vi "AdaptToInputs.vi"(0 "XRef":T25, 1 "Term Types":T22, 2 "State In":T2={"BlockNodeState"={"Terminal Data"=[], "Instance Name"="", "Type Name"="", "Draw Style"=0, "Connector Pane Pattern"=0, "Flags"=0, "Grown Terminal List Order"=[], "Image"={"image type"=0, "image depth"=0, "image"=[], "mask"=[], "colors"=[], "Rectangle"={"left"=0, "top"=0, "right"=0, "bottom"=0}}}, "stateInfo"={"Data storage parameters"={"Name"="", "Format"="TDM", "Connection string"="", "use default"=TRUE}, "Object type"="root", "Selected properties"=[], "Object definitions"=[], "Refnum input wired"=enum."<none>", "Parent object type"="", "Parent object child property"="", "Channel options"=enum."Replace values at index", "PendingCommand"=enum."<none>", "Node style"=enum."Classic", "Only child objects"=FALSE, "TermSpecs"=[], "objectTypeWired"="", "Dynamic format"=FALSE, "Overwrite options"=enum."open or create", "Parameters"=variant, "Format"="", "Node type"=enum."UPDATE", "ImplicitExplicit"=enum."explicit", "Channel type"=enum."Waveform", "Use object with same name"=FALSE, "Show channel terminal"=FALSE, "LabVIEW Version"="", "DataTerminals"=enum."Express", "Size to text"=FALSE, "selected nodes in"=[]}} {"BlockNodeState"."Draw Style" items=["FunctionBlock", "ExpressVI", "Variable", "Elemental I/O", "32x32 Icon", "FunctionBlockCompact"]; "BlockNodeState"."Terminal Data"."Terminal Flags" format="%.0b"}) -> (14 "Reply":T20, 15 "State Out":T2={"BlockNodeState"={"Terminal Data"=[], "Instance Name"="", "Type Name"="", "Draw Style"=0, "Connector Pane Pattern"=0, "Flags"=0, "Grown Terminal List Order"=[], "Image"={"image type"=0, "image depth"=0, "image"=[], "mask"=[], "colors"=[], "Rectangle"={"left"=0, "top"=0, "right"=0, "bottom"=0}}}, "stateInfo"={"Data storage parameters"={"Name"="", "Format"="TDM", "Connection string"="", "use default"=TRUE}, "Object type"="root", "Selected properties"=[], "Object definitions"=[], "Refnum input wired"=enum."<none>", "Parent object type"="", "Parent object child property"="", "Channel options"=enum."Replace values at index", "PendingCommand"=enum."<none>", "Node style"=enum."Classic", "Only child objects"=FALSE, "TermSpecs"=[], "objectTypeWired"="", "Dynamic format"=FALSE, "Overwrite options"=enum."open or create", "Parameters"=variant, "Format"="", "Node type"=enum."UPDATE", "ImplicitExplicit"=enum."explicit", "Channel type"=enum."Waveform", "Use object with same name"=FALSE, "Show channel terminal"=FALSE, "LabVIEW Version"="", "DataTerminals"=enum."Express", "Size to text"=FALSE, "selected nodes in"=[]}} {"BlockNodeState"."Draw Style" items=["FunctionBlock", "ExpressVI", "Variable", "Elemental I/O", "32x32 Icon", "FunctionBlockCompact"]; "BlockNodeState"."Terminal Data"."Terminal Flags" format="%.0b"})   [LabVIEW 2017, in "Open Data Storage.xnode"]
uses:
  <vilib>/Platform/storage/lvStorage.llb/xStorage/Open Data Storage/Open Data Storage.xnode
  <vilib>/XNodeSupport/XNodeXNodeRef.ctl
  <vilib>/XNodeSupport/XNodeTermTypeIDPairs.ctl
  <vilib>/XNodeSupport/XNodeTermTypeIDPair.ctl
  <vilib>/XNodeSupport/XNodeType.ctl
  <vilib>/XNodeSupport/XNodeString.ctl
  <vilib>/Platform/storage/lvStorage.llb/xStorage/Open Data Storage/State.ctl
  <vilib>/BlockNodeSupport/BlockNodeState.ctl
  <vilib>/BlockNodeSupport/TerminalData.ctl
  <vilib>/picture/picture.llb/imagedata.ctl
  <vilib>/Platform/storage/lvStorage.llb/dataStorageParams.ctl
  <vilib>/Platform/storage/lvStorage.llb/_selectedProp.ctl
  <vilib>/Platform/storage/lvStorage.llb/dataModel.ctl
  <vilib>/Platform/storage/Storage.llb/usiTypeDef.ctl
  <vilib>/Platform/storage/Storage.llb/usiPropDef.ctl
  <vilib>/express/express shared/ex_EditUserDefinedProperties/usiDataType.ctl
  <vilib>/Platform/storage/Storage.llb/specialProperties.ctl
  <vilib>/Platform/storage/Storage.llb/usiOverwriteOptions.ctl
  <vilib>/Platform/storage/lvStorage.llb/TerminalDef.ctl
  <vilib>/Platform/storage/lvStorage.llb/_TerminalStyle.ctl
  <vilib>/Utility/XNodeSupport.llb/XRect32.ctl
  <vilib>/Platform/storage/Storage.llb/usiSequenceRepresentation.ctl
  <vilib>/Platform/storage/lvStorage.llb/channelType.ctl
  <vilib>/Platform/storage/lvStorage.llb/_dataTerminals.ctl
  <vilib>/XNodeSupport/XNodeStringArray.ctl
  <vilib>/XNodeSupport/NI_XNodeSupport.lvlib
panel:
  in  "Node type":T1(ring)=enum."CREATE CHILD"
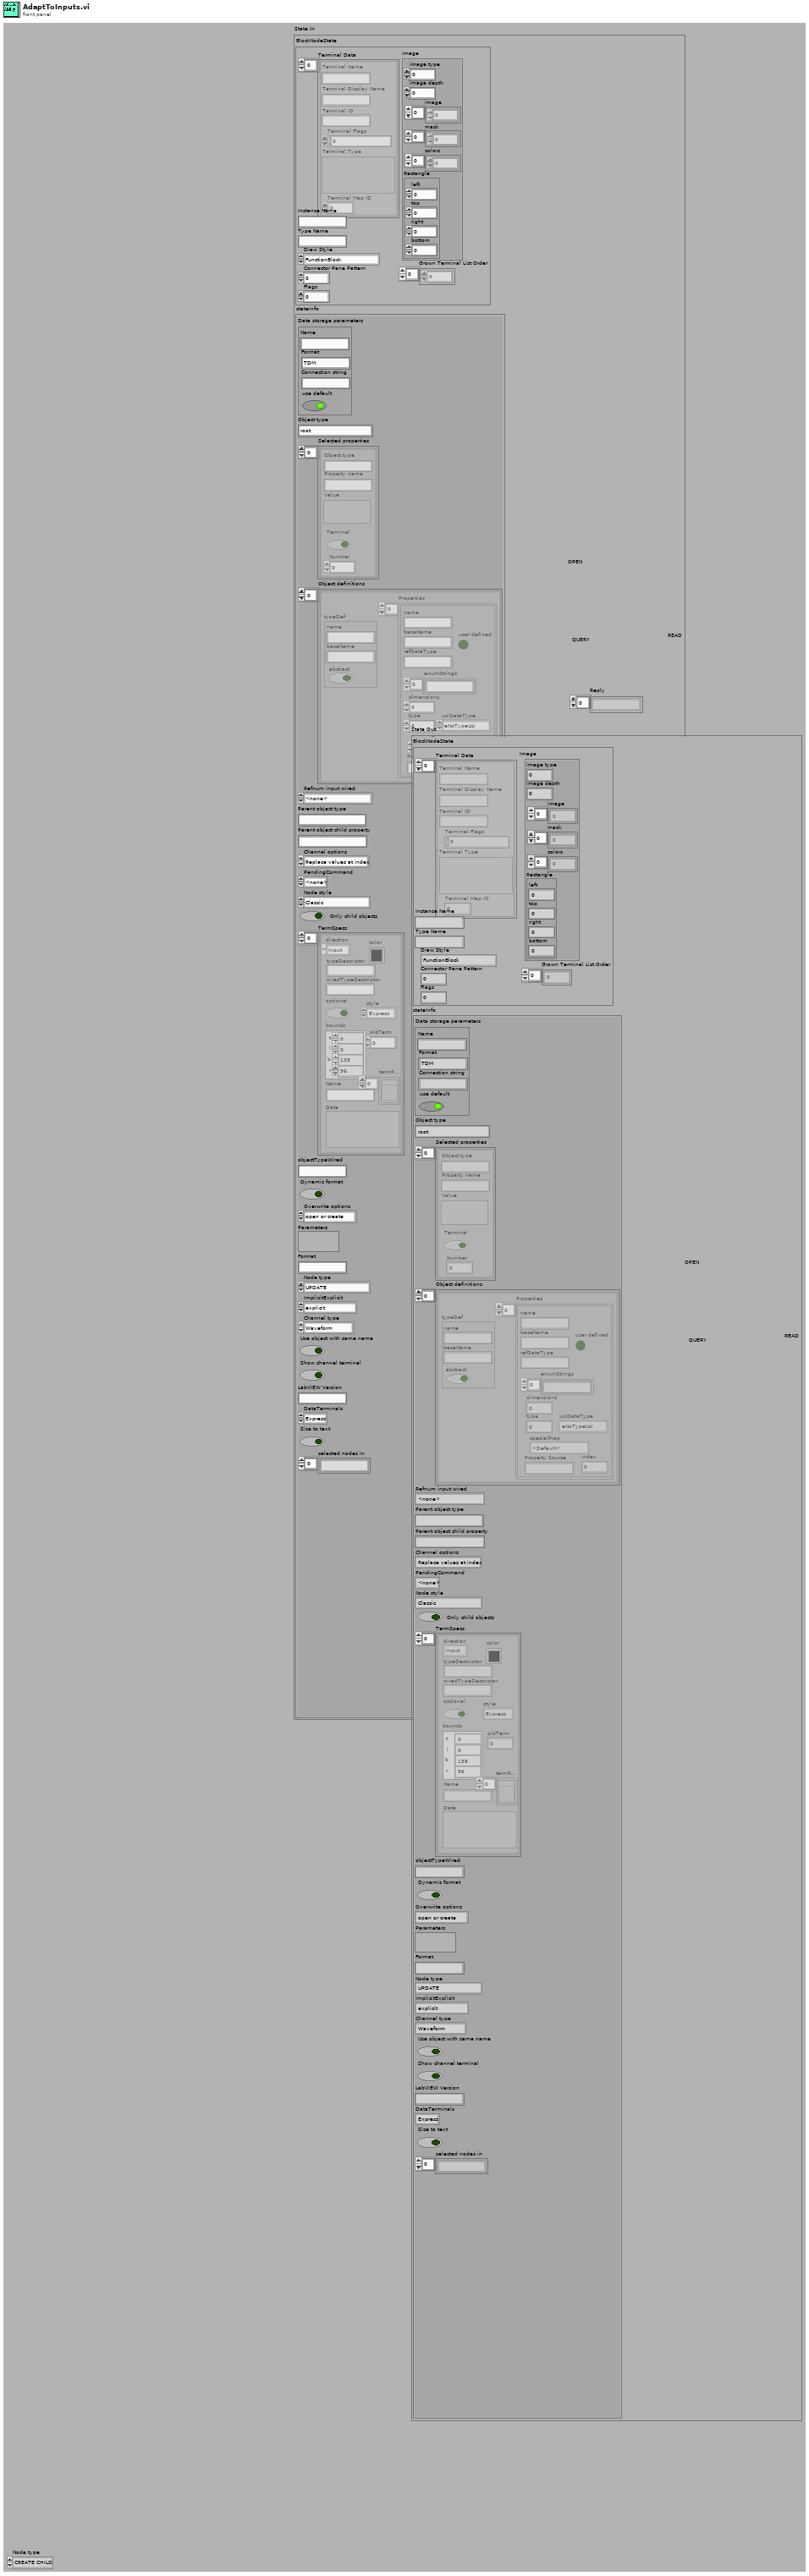
[diagram p1: front panel]
types:
  T1 = enum16{"UPDATE", "READ", "QUERY", "CREATE CHILD", "CREATE", "CONNECT", "DISCONNECT"}
  T2 = typedef "Open Data Storage.xnode/State.ctl" = cluster{"BlockNodeState":T3, "stateInfo":cluster{"Data storage parameters":T6, "Object type":string, "Selected properties":T7[], "Object definitions":T8[], "Refnum input wired":enum16{"Storage", "Generic object", "Typed object", "<none>"}, "Parent object type":string, "Parent object child property":string, "Channel options":T13, "PendingCommand":enum16{"<none>", "SelPopUp", "Init"}, "Node style":enum16{"Classic", "Express"}, "Only child objects":bool, "TermSpecs":T14[], "objectTypeWired":string, "Dynamic format":bool, "Overwrite options":enum16{"open", "open or create", "create or replace", "create", "open (read only)"}, "Parameters":variant, "Format":string, "Node type":enum16{"UPDATE", "READ", "QUERY", "CREATE CHILD", "CREATE", "CONNECT", "DISCONNECT"}, "ImplicitExplicit":T17, "Channel type":T18, "Use object with same name":bool, "Show channel terminal":bool, "LabVIEW Version":string, "DataTerminals":T19, "Size to text":bool, "selected nodes in":string[]}}
  T3 = typedef "BlockNodeState.ctl" = cluster{"Terminal Data":T4[], "Instance Name":string, "Type Name":string, "Draw Style":i32, "Connector Pane Pattern":i32, "Flags":i32, "Grown Terminal List Order":i32[], "Image":T5}
  T4 = typedef "TerminalData.ctl" = cluster{"Terminal Name":string, "Terminal Display Name":string, "Terminal ID":string, "Terminal Flags":i32, "Terminal Type":variant, "Terminal Map ID":i32}
  T5 = typedef "imagedata.ctl" = cluster{"image type":i32, "image depth":i32, "image":u8[], "mask":u8[], "colors":u32[], "Rectangle":cluster{"left":i16, "top":i16, "right":i16, "bottom":i16}}
  T6 = typedef "dataStorageParams.ctl" = cluster{"Name":string, "Format":string, "Connection string":string, "use default":bool}
  T7 = typedef "_selectedProp.ctl" = cluster{"Object type":string, "Property name":string, "Value":variant, "Terminal":bool, "Number":i32}
  T8 = typedef "dataModel.ctl" = cluster{"typeDef":T9, "Properties":T10[]}
  T9 = typedef "usiTypeDef.ctl" = cluster{"name":string, "baseName":string, "abstract":bool}
  T10 = typedef "usiPropDef.ctl" = cluster{"name":string, "baseName":string, "refDataType":string, "dimensions":i32, "type":i32, "user defined":bool, "enumStrings":string[], "usiDataType":T11, "specialProp":T12, "Property Source":string, "index":i32}
  T11 = typedef "usiDataType.ctl" = enum16{"eNoTypeUsi", "eInt8Usi", "eInt16Usi", "eInt32Usi", "eInt64Usi", "eUInt8Usi", "eUInt16Usi", "eUInt32Usi", "eUInt64Usi", "eFloat32Usi", "eFloat64Usi", "- 0", "- 1", "- 2", "- 3", "- 4", "- 5", "- 6", "- 7", "- 8", "- 9", "eString8Usi", "eString16Usi", "eStringUsi", "eEnumUsi", "- 10", "- 11", "- 12", "- 13", "- 14", "eTimeUsi", "- 15", "- 16", "- 17", "- 18", "- 19", "- 20", "- 21", "- 22", "- 23", "eInstanceUsi", "eStoreUsi"}
  T12 = typedef "specialProperties.ctl" = enum16{"<Default>", "Channel Values", "AppendReplace", "ChannelFlags", "ValueFlags", "ImplicitExplicit", "InsertIndex", "ValuesCount", "ComparisonOperator", "Cluster", "DAQmx Channel"}
  T13 = typedef "usiOverwriteOptions.ctl" = enum16{"Append values", "Replace values at index", "Replace all values", "Append if timeline aligns"}
  T14 = typedef "TerminalDef.ctl" = cluster{"direction":enum16{"Input", "Output"}, "typeDescriptor":string, "color":u32, "oldTerm":i32, "style":T15, "optional":bool, "bounds":T16, "termRefs":refnum<vi>[], "Name":string, "Data":variant, "wiredTypeDescriptor":string}
  T15 = typedef "_TerminalStyle.ctl" = enum16{"Express", "Collapsed", "Internal"}
  T16 = typedef "XRect32.ctl" = cluster{"t":i32, "l":i32, "b":i32, "r":i32}
  T17 = typedef "usiSequenceRepresentation.ctl" = enum16{"explicit", "implicit"}
  T18 = typedef "channelType.ctl" = enum16{"Waveform", "Array of Double", "Array of String", "DDT", "Array of UInt8", "Array of Int16", "Array of Int32", "Array of Single", "Array of DateTime", "Array of Waveform", "none", "DateTime", "String", "Double", "Single", "UInt8", "Int16", "Int32"}
  T19 = typedef "_dataTerminals.ctl" = enum16{"Express", "Cluster"}
  T20 = typedef "NI_XNodeSupport.lvlib/XNodeStringArray.ctl" = T21[]
  T21 = typedef "NI_XNodeSupport.lvlib/XNodeString.ctl" = string
  T22 = typedef "NI_XNodeSupport.lvlib/XNodeTermTypeIDPairs.ctl" = T23[]
  T23 = typedef "NI_XNodeSupport.lvlib/XNodeTermTypeIDPair.ctl" = cluster{"Type":T24, "Id":T21}
  T24 = typedef "NI_XNodeSupport.lvlib/XNodeType.ctl" = variant
  T25 = typedef "NI_XNodeSupport.lvlib/XNodeXNodeRef.ctl" = refnum<vi>
  T26 = cluster{"Data storage parameters":T6, "Object type":string, "Selected properties":T7[], "Object definitions":T8[], "Refnum input wired":enum16{"Storage", "Generic object", "Typed object", "<none>"}, "Parent object type":string, "Parent object child property":string, "Channel options":T13, "PendingCommand":enum16{"<none>", "SelPopUp", "Init"}, "Node style":enum16{"Classic", "Express"}, "Only child objects":bool, "TermSpecs":T14[], "objectTypeWired":string, "Dynamic format":bool, "Overwrite options":enum16{"open", "open or create", "create or replace", "create", "open (read only)"}, "Parameters":variant, "Format":string, "Node type":enum16{"UPDATE", "READ", "QUERY", "CREATE CHILD", "CREATE", "CONNECT", "DISCONNECT"}, "ImplicitExplicit":T17, "Channel type":T18, "Use object with same name":bool, "Show channel terminal":bool, "LabVIEW Version":string, "DataTerminals":T19, "Size to text":bool, "selected nodes in":string[]}
  T27 = typedef "_stateInfoWriteProps.ctl" = cluster{"Data storage parameters":T6, "Object type":string, "Selected properties":T7[], "Object definitions":T8[], "Refnum input wired":enum16{"Storage", "Generic object", "Typed object", "<none>"}, "Parent object type":string, "Parent object child property":string, "Channel options":T13, "PendingCommand":enum16{"<none>", "SelPopUp", "Init"}, "Node style":enum16{"Classic", "Express"}, "Only child objects":bool, "TermSpecs":T14[], "objectTypeWired":string, "Dynamic format":bool, "Overwrite options":enum16{"open", "open or create", "create or replace", "create", "open (read only)"}, "Parameters":variant, "Format":string, "Node type":enum16{"UPDATE", "READ", "QUERY", "CREATE CHILD", "CREATE", "CONNECT", "DISCONNECT"}, "ImplicitExplicit":T17, "Channel type":T18, "Use object with same name":bool, "Show channel terminal":bool, "LabVIEW Version":string, "DataTerminals":T19, "Size to text":bool, "selected nodes in":string[]}
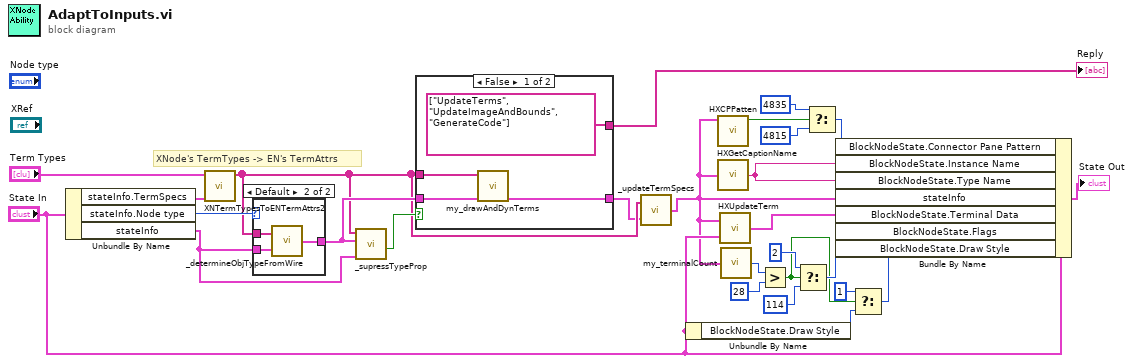
[diagram p0: block diagram]
diagram:
  # "XNode's TermTypes -> EN's TermAttrs"
  n1 = Unbundle By Name("State In") -> ("stateInfo.TermSpecs"=w15:T14[], "stateInfo.Node type"=w16:T1, "stateInfo"=w14:T26)
  n2 = call <vilib>:"XNTermTypesToENTermAttrs2.vi"("EN's termspec"=w15, "XN's term"="Term Types") -> ("Array"=w3:string[])  [unwired: 7 in]
  n3 = case shown="Default" w16 {
    tunnel: [w28 w31] -> w17
    tunnel: w14 -> [w28 w30]
    tunnel: w3 -> [_ w29]
    frame "CONNECT" {
    }
    frame Default {
      n4 = call <vilib>:"_determineObjTypeFromWire.vi"("stateInfoUSIConnect in"=w30, "termAttrs"=w29) -> ("stateInfoUSIConnect out"=w31:T27)
    }
  }
  n5 = call <vilib>:"_supressTypeProp.vi"("stateInfoUSIConnect 2"=w14, "stateInfoUSIConnect 1"=w17, "termAttrs"=w3) -> ("SuppressTypeProp"=w18:bool)  [unwired: 4 in]
  n6 = case shown="False" w18 {
    tunnel: w17 -> [w35 w36]
    tunnel: w3 -> [w34 _]
    tunnel: [string[] ["UpdateTerms", "UpdateImageAndBounds", "GenerateCode"] _] -> w27
    tunnel: [w32 w36] -> w2
    frame False {
      n7 = call <vilib>:"my_drawAndDynTerms.vi"("state in"=w35, "termAttrs"=w34) -> ("state out"=w32:T27)  [unwired: 9 in]
    }
    frame True {
    }
  }
  "Reply" <- w27
  n8 = call <vilib>:"_updateTermSpecs.vi"("stateInfo in"=w2, "termAttrs"=w3) -> ("stateInfo out"=w1:T27)
  n9 = Unbundle By Name("State In") -> ("BlockNodeState.Draw Style"=w6:i32)
  n10 = call <vilib>:"HXCPPatten.vi"("stateInfo"=w1) -> ("x .or. y?"=w21:bool)  [unwired: 10 in]
  n11 = call <vilib>:"HXGetCaptionName.vi"("stateInfoUSIConnect out"=w1) -> ("String"=w20:string)
  n12 = call <vilib>:"HXUpdateTerm.vi"("HX State Info"="State In", "XNode State Info"=w1) -> ("BlockNodeState.Terminal Data"=w24:T4[])
  n13 = call <vilib>:"my_terminalCount.vi"("stateInfo in"=w1) -> ("terminal count"=w13:i32)
  n14 = Greater?(x=w13, y=28) -> (0:w7:bool)
  n15 = Select(t=2, s=w7, f=114) -> (s? t:f=w9:i32)
  n16 = Select(t=4835, s=w21, f=4815 ("t")) -> (s? t:f=w19:i32)
  n17 = Select(t=1, s=w7, f=w6) -> (s? t:f=w4:i32)
  n18 = Bundle By Name(cluster="State In", "BlockNodeState.Connector Pane Pattern"=w19, "BlockNodeState.Instance Name"=w20, "BlockNodeState.Type Name"=w20, "stateInfo"=w1, "BlockNodeState.Terminal Data"=w24, "BlockNodeState.Flags"=w9, "BlockNodeState.Draw Style"=w4) -> (→"State Out":T2)
